vi "Main.vi"(11 "Module Admin":refnum<class "Delacor_lib_QMH_Module Admin.lvclass">) -> ()   [LabVIEW 2020, in "Acquisition.lvlib"]
doc: "This template is based off of the Queued Message Handler design pattern and the Queued Message Handler project template that ships with LabVIEW.\n\nThe main difference is that the queue is private to this module and communication between modules is performed via Broadcast and Request events.\n\nRequest events are wrapped in public API methods and are handled in the Event Handling Loop (EHL) of this VI. Any module can register for Broadcast events sent by this module. The EHL generates messages based on user interface actions.\n\nThe Message Handling Loop (MHL) processes messages generated by the EHL, or by other messages. The messages are string values, so new messages can be added easily to the Message Cases case structure in the MHL. Each message cluster can also provide an optional value for Message Data, which is a variant that can be converted to whatever message-specific data is required.\n_____\nBased on Delacor QMH Project Template 4.0.0.47.\n_____\nBased on DQMH Project Template 6.0.0.91."
uses:
  Acquisition.lvlib
  <vilib>/Delacor/Delacor QMH/Libraries/Module Admin_class/Delacor_lib_QMH_Module Admin.lvclass
  Module Data--cluster.ctl
  CML Shared/Signal Type--enum.ctl
  CML Shared/Calibration Values--cluster.ctl
  Stop Argument--cluster.ctl
  <vilib>/Delacor/Delacor QMH/Libraries/Message Queue_class/Delacor_lib_QMH_Message Queue.lvclass/Delacor_lib_QMH_Message Queue.ctl
  <vilib>/Delacor/Delacor QMH/Libraries/Module Admin_class/Delacor_lib_QMH_Module Admin.lvclass/Delacor_lib_QMH_Module Admin.ctl
  Start Acquiring Argument--cluster.ctl
  Start Acquiring (Reply Payload)--cluster.ctl
  Stop Acquiring Argument--cluster.ctl
  Settings Editor/Update Application Settings (Reply Payload)--cluster.ctl
  Settings Editor/Settings--cluster.ctl
  <vilib>/Utility/miscctls.llb/LVPointTypeDef.ctl
  <vilib>/Delacor/Delacor QMH/Libraries/Message Queue_class/Delacor_lib_QMH_Enqueue Message (Single).vi
  <vilib>/Delacor/Delacor QMH/Libraries/Module Admin_class/Delacor_lib_QMH_Get External Launch.vi
  <vilib>/Utility/error.llb/Error Cluster From Error Code.vi
  <vilib>/ErrorRing/Error Ring.xnode
  <vilib>/Delacor/Delacor QMH/Libraries/Message Queue_class/Delacor_lib_QMH_Message Queue.lvclass
  CML Shared/CML Shared.lvlib
  Settings Editor/Settings Editor.lvlib
  Logger/Logger.lvlib
panel:
  out "Settings":T1
  out "Graph Data":waveform(dbl)[](array[waveform])
  out "error out":errorcluster
  # "This is a headless module. Show its panel to confirm that the Settings are updated correctly and other debugging tasks. Use the Settings Editor to change the settings for this module."
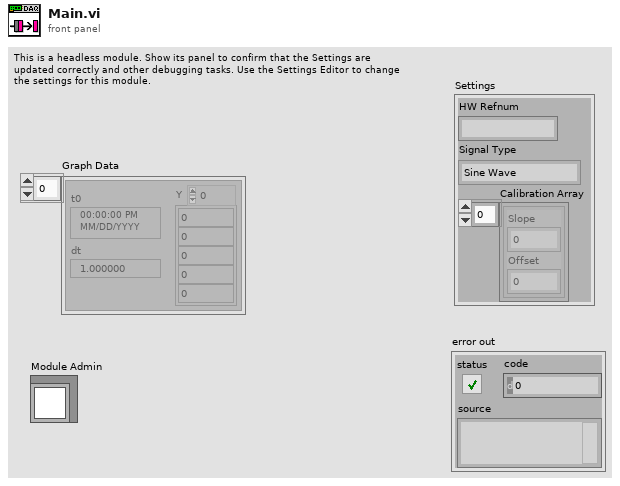
[diagram p1: front panel]
types:
  T1 = typedef "Acquisition.lvlib/Module Data--cluster.ctl" = cluster{"HW Refnum":string, "Signal Type":T2, "Calibration Array":T3[]}
  T2 = typedef "CML Shared.lvlib/Signal Type--enum.ctl" = enum16{"Sine Wave", "Square with Noise"}
  T3 = typedef "CML Shared.lvlib/Calibration Values--cluster.ctl" = cluster{"Slope":dbl, "Offset":dbl}
  T4 = typedef "Settings Editor.lvlib/Broadcast Events--cluster.ctl" = cluster{"Module Did Init":refnum<user-event>, "Status Updated":refnum<user-event>, "Error Reported":refnum<user-event>, "Module Did Stop":refnum<user-event>, "Update Module Execution Status":refnum<user-event>, "Application Settings Updated":refnum<user-event>}
  T5 = typedef "Acquisition.lvlib/Request Events--cluster.ctl" = cluster{"Stop Module":refnum<user-event>, "Show Panel":refnum<user-event>, "Hide Panel":refnum<user-event>, "Get Module Execution Status":refnum<user-event>, "Show Diagram":refnum<user-event>, "Stop Acquiring":refnum<user-event>, "Wakeup Helper Loop":refnum<user-event>, "Change Settings":refnum<user-event>, "Calibrate DAQ":refnum<user-event>, "Start Acquiring":refnum<user-event>}
  T6 = enum32{"invalid lock state", "Not Locked", "Locked (No Password)", "Password-protected"}
  T7 = typedef "Acquisition.lvlib/Stop Argument--cluster.ctl" = cluster{"Origin":string, "Exit via Stop Module Req?":bool, "Wait for Module to stop?":bool}
  T8 = typedef "Acquisition.lvlib/Start Acquiring Argument--cluster.ctl" = cluster{"Wait Notifier":refnum<notifier>, "wait for reply":bool}
  T9 = typedef "Acquisition.lvlib/Stop Acquiring Argument--cluster.ctl" = cluster{"Boolean":bool}
  T10 = typedef "Settings Editor.lvlib/Update Application Settings (Reply Payload)--cluster.ctl" = cluster{"Settings":T11, "Update Settings_error":errorcluster}
  T11 = typedef "Settings Editor.lvlib/Settings--cluster.ctl" = cluster{"Signal Type":T2, "Calibration Array":T3[], "Log File Base Path":path}
  T12 = typedef "LVPointTypeDef.ctl" = cluster{"Horizontal":i16, "Vertical":i16}
  T13 = enum32{"Invalid", "Standard", "Closed", "Hidden", "Minimized", "Maximized"}
  T14 = typedef "Acquisition.lvlib/Start Acquiring (Reply Payload)--cluster.ctl" = cluster{"HW ID":string, "Start Acquiring_error":errorcluster}
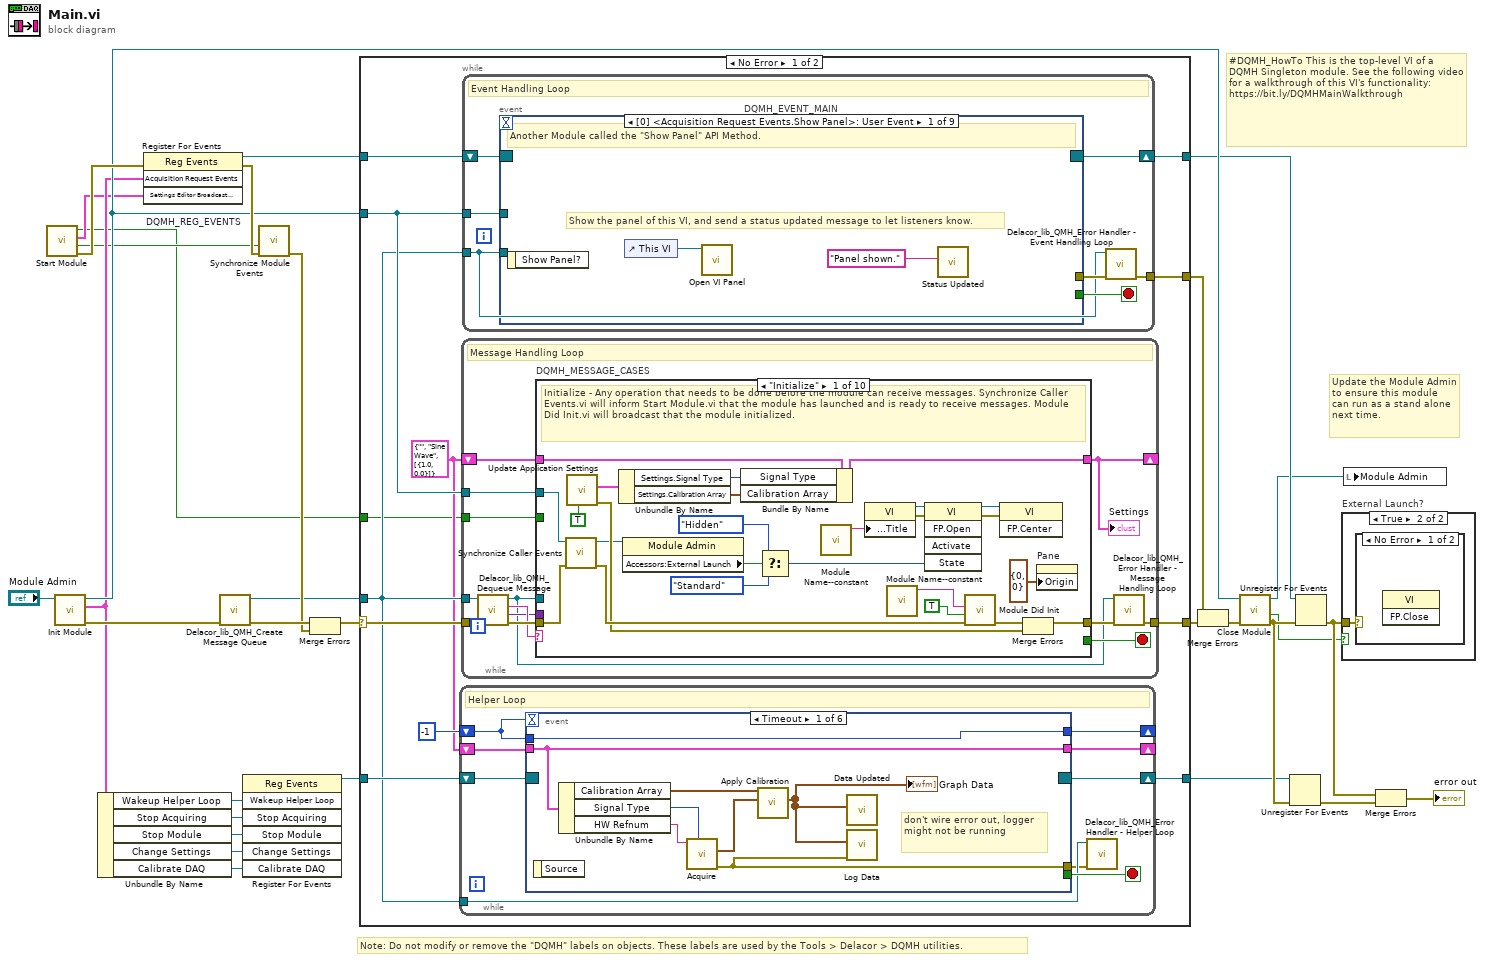
[diagram p0: block diagram]
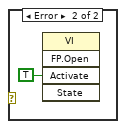
[diagram p3: hidden frame]
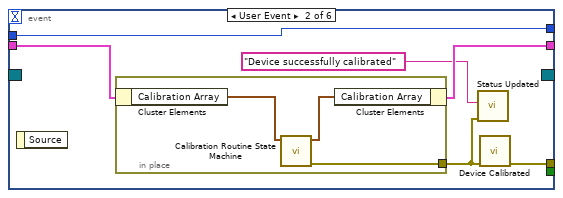
[diagram p4: hidden frame]
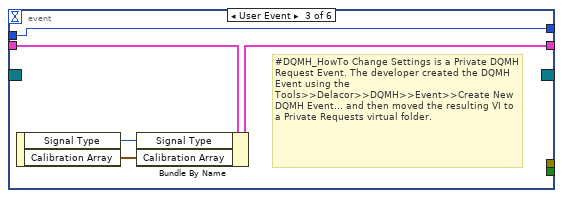
[diagram p5: hidden frame]
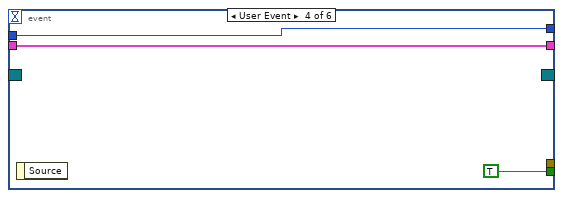
[diagram p6: hidden frame]
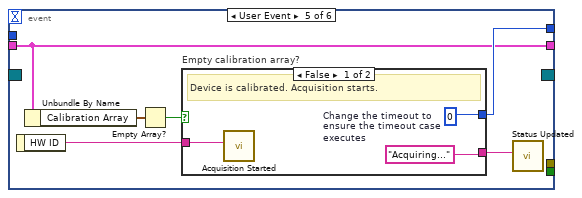
[diagram p7: hidden frame]
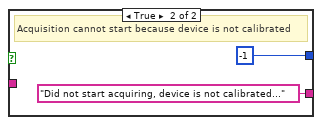
[diagram p8: hidden frame]
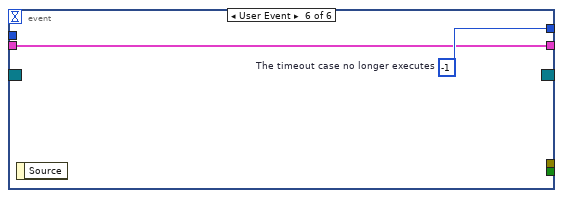
[diagram p9: hidden frame]
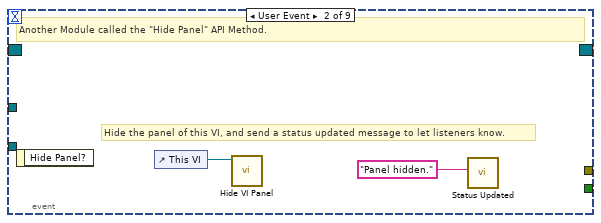
[diagram p10: hidden frame]
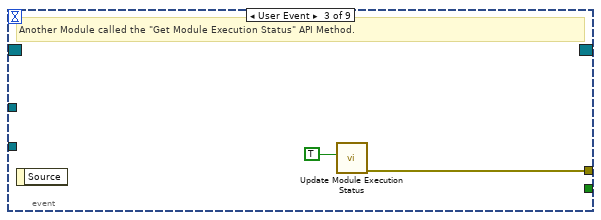
[diagram p11: hidden frame]
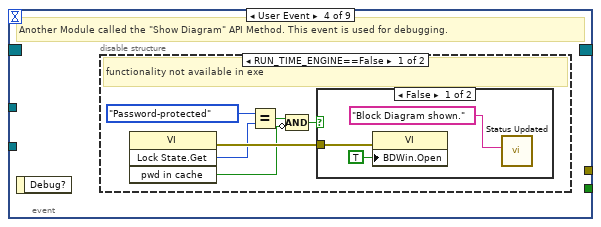
[diagram p12: hidden frame]
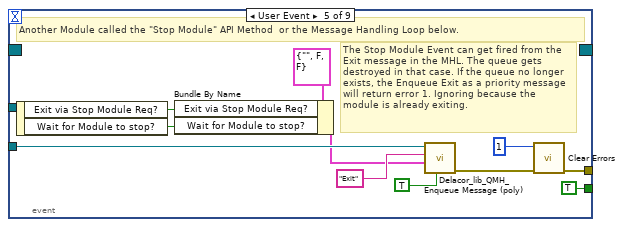
[diagram p15: hidden frame]
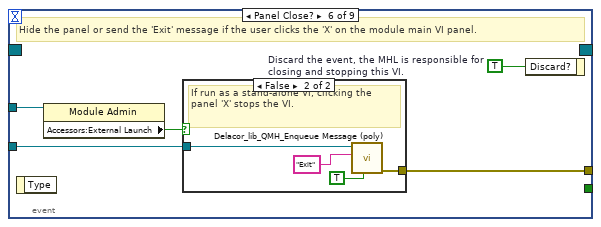
[diagram p16: hidden frame]
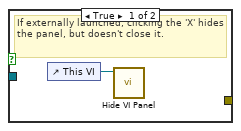
[diagram p17: hidden frame]
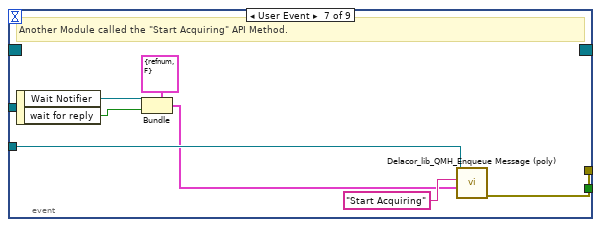
[diagram p18: hidden frame]
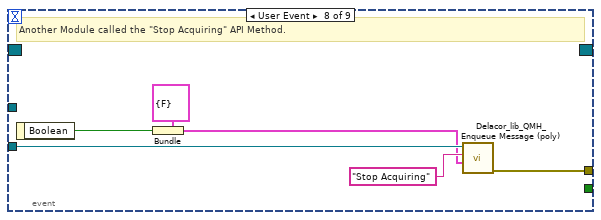
[diagram p19: hidden frame]
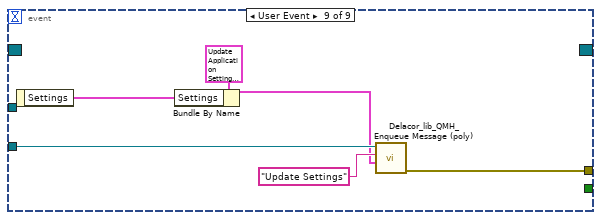
[diagram p20: hidden frame]
diagram:
  # "#DQMH_HowTo This is the top-level VI of a DQMH Singleton module. See the following video for a walkthrough of this VI's functionality: https://bit.ly/DQMHMainWalkthrough"
  # "Note: Do not modify or remove the \"DQMH\" labels on objects. These labels are used by the Tools > Delacor > DQMH utilities."
  # "Update the Module Admin to ensure this module can run as a stand alone next time."
  n1 = call "Start Module.vi"() -> ("error out"=w24:errorcluster, "Wait for Event Sync?"=w5:bool, "Settings Editor Broadcast Events"=w6:T4, "Module Was Already Running?"=w1:bool)  [unwired: 8 in]
  n2 = call "Init Module.vi"("Singleton Module Admin in"="Module Admin") -> ("error out"=w30:errorcluster, "Acquisition Request Events"=w11:T5, "Singleton Module Admin out"=w18:refnum<class "Delacor_lib_QMH_Module Admin.lvclass">)  [unwired: 8 in]
  n3 = Unbundle By Name(w11) -> ("Wakeup Helper Loop"=w7:refnum<user-event>, "Stop Acquiring"=w10:refnum<user-event>, "Stop Module"=w9:refnum<user-event>, "Change Settings"=w4:refnum<user-event>, "Calibrate DAQ"=w3:refnum<user-event>)
  n4 = register-events "DQMH_REG_EVENTS"(error in=w24, w11, w6) -> (reference out=w16:refnum<event-registration>, error out=w23:errorcluster)  [unwired: 1 in]
  n5 = call <vilib>:"Delacor_lib_QMH_Create Message Queue.vi"("error in"=w30) -> ("error out"=w26:errorcluster, "Message Queue"=w15:refnum<class "Delacor_lib_QMH_Message Queue.lvclass">)  [unwired: 9 in]
  n6 = register-events(w7, w10, w9, w4, w3) -> (reference out=w8:refnum<event-registration>)  [unwired: 2 in, 1 out]
  n7 = call "Synchronize Module Events.vi"("error in (no error)"=w23, "Wait for Event Sync?"=w5) -> ("error out"=w22:errorcluster)  [unwired: 9 in]
  n8 = Merge Errors(w26, w22) -> (w25:errorcluster)
  n9 = case shown="No Error" w25 {
    selector: w25 -> [w41 w286]
    tunnel: [w43 w285] -> w31
    tunnel: [w40 w294] -> w17
    tunnel: w16 -> [w39 w294]
    tunnel: w15 -> [w35 w287]
    tunnel: [w42 _] -> w29
    tunnel: w18 -> [w38 w290]
    tunnel: w8 -> [w36 w289]
    tunnel: [w33 w289] -> w2
    tunnel: w1 -> [w32 w288]
    frame No Error {
      w34 = T1 {"HW Refnum"="", "Signal Type"=enum."Sine Wave", "Calibration Array"=[{"Slope"=1.0, "Offset"=0.0}]} ("Data Cluster")
      n10 = while {
        shift-right: [w52] -> _
        shift-left: -1 -> [w51]
        tunnel: w35 -> [w45]
        shift-right: [w48] -> _
        shift-left: w34 -> [w47]
        shift-right: [w46] -> w33
        shift-left: w36 -> [w50]
        stop <- w49 stop-if-true
        # "Helper Loop"
        n11 = event shown="[0] Timeout" {
          selector: w50 -> [_ _ _ _ _ _]
          dyn-events: [_ _ _ _ _ _] -> w46
          timeout: w51 -> [_ _ _ _ _ _]
          tunnel: [w59 w65 w74 w77 w82 w90] -> w52
          tunnel: w51 -> [w59 w65 w74 w77 _ _]
          tunnel: [_ _ _ TRUE _ _] -> w49
          tunnel: [w60 w66 _ _ _ _] -> w44
          tunnel: [w56 w63 w72 w75 w79 w89] -> w48
          tunnel: w47 -> [w56 w64 w73 w75 w79 w89]
          event Timeout {
            # "don't wire error out, logger might not be running"
            n12 = event-data() -> ()  [unwired: 1 in, 1 out]
            n13 = Unbundle By Name(w56) -> ("Calibration Array"=w54:T3[], "Signal Type"=w58:T2, "HW Refnum"=w57:string)
            n14 = call "Acquire.vi"("Signal Type"=w58, "HW ID in"=w57) -> ("error out"=w60:errorcluster, "Graph Data"=w55:waveform(dbl)[])  [unwired: 7 in, 1 out]
            n15 = call "Apply Calibration.vi"("Graph Data"=w55, "Calibration Array"=w54) -> ("Calibrated Data"=w53:waveform(dbl)[])  [unwired: 9 in]
            "Graph Data" <- w53
            n16 = call "Data Updated.vi"("Graph Data"=w53) -> ()  [unwired: 10 in, 1 out]
            n17 = call "Log Data.vi"("error in (no error)"=w60, "Waveforms"=w53) -> ()  [unwired: 9 in, 1 out]
          }
          event User Event {
            n18 = event-data() -> ()  [unwired: 1 in, 1 out]
            n19 = in-place {
              in-place-border: [w69] -> w62
              n20 = in-place-cluster #1(w64) -> ("Calibration Array"=w68:T3[])
              n21 = call "Calibration Routine State Machine.vi"("Calibration Array in"=w68) -> ("error out"=w69:errorcluster, "Calibration Array out"=w67:T3[])  [unwired: 9 in]
              n22 = in-place-cluster #1("Calibration Array"=w67) -> (w63:T1)
            }
            n23 = call "Status Updated.vi"("error in (no error)"=w62, "Status"="Device successfully calibrated") -> ()  [unwired: 9 in, 1 out]
            n24 = call "Device Calibrated.vi"("error in (no error)"=w62) -> ("error out"=w66:errorcluster)  [unwired: 10 in]
          }
          event User Event {
            # "#DQMH_HowTo Change Settings is a Private DQMH Request Event. The developer created the DQMH Event using the Tools>>Delacor>>DQMH>>Event>>Create New DQMH Event... and then moved the resulting VI to a Private Requests virtual folder."
            n25 = event-data() -> ("Signal Type"=w71:T2, "Calibration Array"=w70:T3[])  [unwired: 1 in]
            n26 = Bundle By Name(cluster=w73, "Signal Type"=w71, "Calibration Array"=w70) -> (w72:T1)
          }
          event User Event {
            n27 = event-data() -> ()  [unwired: 1 in, 1 out]
          }
          event User Event {
            n28 = event-data() -> ("HW ID"=w80:string)  [unwired: 1 in]
            n29 = Unbundle By Name(w79) -> ("Calibration Array"=w78:T3[])
            n30 = Empty Array?(array=w78) -> (empty?=w83:bool)
            n31 = case "Empty calibration array?" shown="False" w83 {
              tunnel: ["Acquiring..." ("Status") "Did not start acquiring, device is not calibrated..." ("Status")] -> w81
              tunnel: [w85 -1] -> w82
              tunnel: w80 -> [w86 _]
              frame False {
                w85 = 0  # Change the timeout to ensure the timeout case executes
                # "Device is calibrated. Acquisition starts."
                n32 = call "Acquisition Started.vi"("HW ID"=w86) -> ()  [unwired: 10 in, 1 out]
              }
              frame True {
                # "Acquisition cannot start because device is not calibrated"
              }
            }
            n33 = call "Status Updated.vi"("Status"=w81) -> ()  [unwired: 10 in, 1 out]
          }
          event User Event {
            w90 = -1  # The timeout case no longer executes
            n34 = event-data() -> ()  [unwired: 1 in, 1 out]
          }
        }
        n35 = call-dynamic "Delacor_lib_QMH_Error Handler - Helper Loop.vi"("error in"=w44, "Message Queue in"=w45) -> ()  [unwired: 8 in, 2 out]
      }
      n36 = while {
        tunnel: w35 -> [w156]
        shift-right: [w160] -> _
        shift-left: w34 -> [w161]
        tunnel: w41 -> [w164]
        tunnel: [w162] -> w43
        tunnel: w38 -> [w154]
        tunnel: w32 -> [w153]
        stop <- w159 stop-if-true
        # "Message Handling Loop"
        n37 = call-dynamic "Delacor_lib_QMH_Dequeue Message.vi"("error in"=w164, "Message Queue in"=w156) -> ("error out"=w163:errorcluster, "Message Data"=w157:variant, "Message"=w158:string, "Message Queue out"=w155:refnum<class "Delacor_lib_QMH_Message Queue.lvclass">)  [unwired: 6 in]
        n38 = case "DQMH_MESSAGE_CASES" shown="\"Initialize\"" w158 {
          selector: w158 -> [_ _ _ _ _ _ _ _ _ w272]
          tunnel: w155 -> [_ _ _ _ _ _ _ w237 w261 _]
          tunnel: w163 -> [w188 w192 w205 w219 w229 w232 w234 w244 w268 w275]
          tunnel: [w185 w192 w203 w217 w221 w231 w234 w240 w265 w276] -> w165
          tunnel: w161 -> [w175 w191 w193 w214 w226 w230 w233 w239 w253 w273]
          tunnel: [w170 w191 w201 w214 w226 w230 w233 w239 w253 w273] -> w160
          tunnel: [_ _ _ _ _ _ _ _ w260 _] -> w159
          tunnel: w157 -> [_ _ w200 w216 w227 _ _ w238 w259 _]
          tunnel: w154 -> [w176 _ _ _ _ _ _ w236 w254 _]
          tunnel: w153 -> [_ _ _ _ _ _ _ _ w251 _]
          frame "Initialize" {
            # "Initialize - Any operation that needs to be done before the module can receive messages. Synchronize Caller Events.vi will inform Start Module.vi that the module has launched and is ready to receive messages. Module Did Init.vi will broadcast that the module initialized."
            n39 = call "Synchronize Caller Events.vi"("error in (no error)"=w188, "Singleton Module Admin in"=w176) -> ("error out"=w187:errorcluster, "Singleton Module Admin out"=w172:refnum<class "Delacor_lib_QMH_Module Admin.lvclass">)  [unwired: 8 in]
            n40 = call "Update Application Settings.vi"("wait for reply (T)"=TRUE) -> ("error out"=w184:errorcluster, "Reply Payload"=w169:T10)  [unwired: 8 in, 1 out]
            n41 = Unbundle By Name(w169) -> ("Settings.Signal Type"=w168:T2, "Settings.Calibration Array"=w167:T3[])
            n42 = property class="Module Admin"(reference=w172) -> ("Accessors:External Launch"=w180:bool)  [unwired: 1 in, 2 out]
            n43 = Bundle By Name(cluster=w175, "Signal Type"=w168, "Calibration Array"=w167) -> (w170:T1)
            n44 = Select(t=T13."Hidden" ("State"), s=w180, f=T13."Standard" ("State")) -> (s? t:f=w177:T13)
            n45 = call "Module Name--constant.vi"() -> ("Module Name"=w183:string)  [unwired: 11 in]
            n46 = property class="VI"("Front Panel.Title"=w183) -> (reference out=w182:refnum<vi>, error out=w190:errorcluster)  [unwired: 2 in]
            n47 = call "Module Name--constant.vi"() -> ("Module Name"=w173:string)  [unwired: 11 in]
            n48 = invoke class="VI" method="FP.Open"(reference=w182, error in=w190, "State"=w177) -> (reference out=w181:refnum<vi>, error out=w189:errorcluster)  [unwired: 2 in, 3 out]
            n49 = call "Module Did Init.vi"("error in (no error)"=w187, "Initialized?"=TRUE, "Origin"=w173) -> ("error out"=w186:errorcluster)  [unwired: 8 in]
            n50 = invoke class="VI" method="FP.Center"(reference=w181, error in=w189) -> ()  [unwired: 1 in, 3 out]
            n51 = Merge Errors(w186, w184) -> (w185:errorcluster)
            n52 = property on="Pane" class="Pane"("Origin"=T12 {"Horizontal"=0, "Vertical"=0}) -> ()  [unwired: 2 in, 2 out]
          }
          frame "---Module Specific---" {
            # "Separator -- The following cases handle messages specific to this Module."
          }
          frame "Start Acquiring" {
            # "Requests Acquisition Module to start acquiring."
            n53 = Variant To Data(error in=w205, type=T8 {"Wait Notifier"=refnum, "wait for reply"=FALSE} ("Start Acquisition Argument"), Variant=w200) -> (data=w198:T8, error out=w202:errorcluster)
            n54 = in-place {
              in-place-border: [w211] -> w204
              in-place-border: w202 -> [w210]
              in-place-border: [w206] -> w194
              n55 = in-place-cluster #2(w193) -> ("HW Refnum"=w207:string)
              n56 = call "Initialize Hardware References.vi"("error in (no error)"=w210, "HW Refnum in"=w207) -> ("error out"=w209:errorcluster, "HW Refnum out"=w208:string)  [unwired: 8 in]
              n57 = call "Configure Hardware.vi"("error in (no error)"=w209, "HW Refnum in"=w208) -> ("error out"=w211:errorcluster, "HW Refnum out"=w206:string)  [unwired: 8 in]
              n58 = in-place-cluster #2("HW Refnum"=w206) -> (w201:T1)
            }
            n59 = Bundle By Name(cluster=T14 {"HW ID"="", "Start Acquiring_error"={"status"=FALSE, "code"=0, "source"=""}} ("Start Acquisition (Reply Payload)"), "HW ID"=w194, "Start Acquiring_error"=w204) -> (w196:T14)
            n60 = Unbundle By Name(w198) -> ("Wait Notifier"=w197:refnum<notifier>)
            n61 = call "Wakeup Helper Loop.vi"("error in (no error)"=w204, "HW ID"=w194) -> ("error out"=w203:errorcluster)  [unwired: 9 in]
            n62 = Send Notification(notification=w196, notifier=w197) -> ()  [unwired: 1 in, 2 out]
          }
          frame "Stop Acquiring" {
            # "Requests the Acquisition Module to stop acquiring"
            n63 = Variant To Data(error in=w219, type=T9 {"Boolean"=FALSE} ("Stop Acquiring Argument"), Variant=w216) -> (error out=w218:errorcluster)  [unwired: 1 out]
            n64 = Unbundle By Name(w214) -> ("HW Refnum"=w213:string)
            n65 = call "Stop Acquisition.vi"("error in (no error)"=w218, "HW Refnum"=w213) -> ("error out"=w217:errorcluster)  [unwired: 9 in]
            n66 = call "Acquisition Stopped.vi"("error in (no error)"=w217) -> ()  [unwired: 10 in, 1 out]
            n67 = call "Status Updated.vi"("error in (no error)"=w217, "Status"="Acquisition Stopped") -> ()  [unwired: 9 in, 1 out]
          }
          frame "Update Settings" {
            # "Send the Change Settings event to the helper loop."
            # "The Settings Editor broadcasted that the settings have changed."
            n68 = Variant To Data(error in=w229, type=T10 {"Settings"={"Signal Type"=enum."Sine Wave", "Calibration Array"=[], "Log File Base Path"=path ""}, "Update Settings_error"={"status"=FALSE, "code"=0, "source"=""}} ("Settings Updated Argument"), Variant=w227) -> (data=w224:T10, error out=w228:errorcluster)
            n69 = Unbundle By Name(w224) -> ("Settings.Signal Type"=w223:T2, "Settings.Calibration Array"=w222:T3[])
            n70 = call "Change Settings.vi"("error in (no error)"=w228, "Calibration Array"=w222, "Signal Type"=w223) -> ("error out"=w221:errorcluster)  [unwired: 8 in]
            n71 = call "Status Updated.vi"("error in (no error)"=w221, "Status"="Settings Updated") -> ()  [unwired: 9 in, 1 out]
          }
          frame "---Copy This Frame---" {
            # "Duplicate this frame when creating new messages.  Change this comment in the duplicated frame to describe this message."
            n72 = Merge Errors(w232) -> (w231:errorcluster)
          }
          frame "---Exit and Error Handling---" {
            # "Separator - The following cases handle errors and exit messages."
          }
          frame "Error" {
            # "Error - Check the error message data and respond accordingly. This message is sent by the \"Error Handler\" VIs at the end of each loop in this application."
            n73 = property class="Module Admin"(reference=w236) -> ("Accessors:External Launch"=w235:bool)  [unwired: 1 in, 2 out]
            n74 = Variant To Data(error in=w244, type=errorcluster {"status"=FALSE, "code"=0, "source"=""} ("error constant"), Variant=w238) -> (data=w245:errorcluster, error out=w242:errorcluster)
            n75 = call "Error Reported.vi"("Error"=w245) -> ()  [unwired: 10 in, 1 out]
            n76 = case shown="False" w235 {
              tunnel: [w250 _] -> w241
              tunnel: w237 -> [w248 _]
              tunnel: w245 -> [w249 _]
              frame False {
                # "If the module is running standalone, then pop up an error dialog and call the \"Exit\" message."
                n77 = call <vilib>:"Simple Error Handler.vi"("error in (no error)"=w249) -> ()  [unwired: 4 in, 5 out]
                n78 = call-poly <vilib>:"Delacor_lib_QMH_Enqueue Message (poly).vi"("Priority Message? (F)"=TRUE, "Message"="Exit", "Message Queue in"=w248) -> ("error out"=w250:errorcluster)  [unwired: 7 in, 1 out]
              }
              frame True {
                # "If the module was launched externally, calling the Error Reported broadcast VI is the only action performed by the \"Error\" message. The module's caller can then process the error appropriately."
              }
            }
            n79 = Merge Errors(w242, w241) -> (w240:errorcluster)
            n80 = local write "error out"(w240) -> ()
          }
          frame "Exit" {
            w258 = 91  # 91: not all Exit messages will have an argument
            w260 = TRUE  # Stop the VI
            # "Release the message queue reference"
            # "Exit - Exit the application."
            n81 = Variant To Data(error in=w268, type=T7 {"Origin"="", "Exit via Stop Module Req?"=FALSE, "Wait for Module to stop?"=FALSE} ("Stop Argument"), Variant=w259) -> (data=w256:T7, error out=w264:errorcluster)
            n82 = call <vilib>:"Clear Errors.vi"("error in (no error)"=w264, "specific error code to clear (0: all)"=w258) -> ("error out"=w267:errorcluster)  [unwired: 4 in, 1 out]
            n83 = Unbundle By Name(w253) -> ("HW Refnum"=w252:string)
            n84 = control-ref of="This VI"() -> (w255:refnum<vi>)
            n85 = call "Handle Exit.vi"("Stop Argument"=w256, "Admin in"=w254, "VI reference"=w255) -> ("error out"=w263:errorcluster)  [unwired: 7 in, 1 out]
            n86 = call "Close Hardware References.vi"("HW Refnum in"=w252) -> ("error out"=w262:errorcluster)  [unwired: 9 in, 1 out]
            n87 = call-dynamic "Delacor_lib_QMH_Release Message Queue.vi"("error in"=w267, "Message Queue"=w261) -> ("error out"=w266:errorcluster)  [unwired: 9 in]
            n88 = case "Settings Editor was\nalready running?" shown="False" w251 {
              frame False {
                n89 = call "Module Name--constant.vi"() -> ("Module Name"=w270:string)  [unwired: 11 in]
                n90 = call "Stop Module.vi"("Wait for Module to Stop? (F)"=TRUE, "Origin"=w270) -> ()  [unwired: 9 in, 1 out]
              }
              frame True {
                # "Another Module is\nin charge of stopping Settings Editor"
              }
            }
            n91 = Merge Errors(w266, w263, w262) -> (w265:errorcluster)
          }
          frame Default {
            # "'Default' case only runs if there is a message that isn't defined in any of the other cases.  Output a programming error."
            n92 = call "Module Name--constant.vi"() -> ("Module Name"=w271:string)  [unwired: 11 in]
            n93 = xnode "Error Ring"("parameter 0"=w272, "parameter 1"=w271) -> ("error out"=w274:errorcluster)
            n94 = Merge Errors(w275, w274) -> (w276:errorcluster)
          }
        }
        "Settings" <- w160
        n95 = call-dynamic "Delacor_lib_QMH_Error Handler - Message Handling Loop.vi"("error in"=w165, "Message Queue in"=w155) -> ("dup error in"=w162:errorcluster)  [unwired: 8 in, 1 out]
      }
      n96 = while {
        tunnel: w35 -> [w91]
        shift-right: [w94] -> w40
        shift-left: w39 -> [w95]
        tunnel: [w96] -> w42
        tunnel: w38 -> [w92]
        stop <- w93 stop-if-true
        # "Event Handling Loop"
        n97 = event "DQMH_EVENT_MAIN" shown="[0] <Acquisition Request Events.Show Panel>: User Event" {
          selector: w95 -> [_ _ _ _ _ _ _ _ _]
          dyn-events: [_ _ _ _ _ _ _ _ _] -> w94
          timeout: _ -> [_ _ _ _ _ _ _ _ _]
          tunnel: [_ _ _ _ TRUE ("Discard?") _ _ _ _] -> w93
          tunnel: w91 -> [_ _ _ _ w119 w126 w140 w145 w150]
          tunnel: [_ _ w103 _ w122 w128 w136 w146 w152] -> w97
          tunnel: w92 -> [_ _ _ _ _ w125 _ _ _]
          event User Event {
            # "Show the panel of this VI, and send a status updated message to let listeners know."
            # "Another Module called the \"Show Panel\" API Method."
            n98 = event-data() -> ()  [unwired: 1 in, 1 out]
            n99 = control-ref of="This VI"() -> (w99:refnum<vi>)
            n100 = call "Open VI Panel.vi"("VI"=w99) -> ()  [unwired: 10 in, 1 out]
            n101 = call "Status Updated.vi"("Status"="Panel shown." ("format string")) -> ()  [unwired: 10 in, 1 out]
          }
          event User Event {
            # "Hide the panel of this VI, and send a status updated message to let listeners know."
            # "Another Module called the \"Hide Panel\" API Method."
            n102 = event-data() -> ()  [unwired: 1 in, 1 out]
            n103 = control-ref of="This VI"() -> (w101:refnum<vi>)
            n104 = call "Hide VI Panel.vi"("VI"=w101) -> ()  [unwired: 10 in, 1 out]
            n105 = call "Status Updated.vi"("Status"="Panel hidden." ("format string")) -> ()  [unwired: 10 in, 1 out]
          }
          event User Event {
            # "Another Module called the \"Get Module Execution Status\" API Method."
            n106 = event-data() -> ()  [unwired: 1 in, 1 out]
            n107 = call "Update Module Execution Status.vi"("Running?"=TRUE) -> ("error out"=w103:errorcluster)  [unwired: 10 in]
          }
          event User Event {
            # "Another Module called the \"Show Diagram\" API Method. This event is used for debugging."
            n108 = event-data() -> ()  [unwired: 1 in, 1 out]
            n109 = disable-structure shown="RUN_TIME_ENGINE==False" {
              frame condition #0 (active) {
                # "functionality not available in exe"
                n110 = invoke class="VI" method="Lock State.Get"() -> (error out=w109:errorcluster, "Get Lock State"=w108:T6, "pwd in cache"=w105:bool)  [unwired: 4 in, 1 out]
                n111 = Equal?(x=T6."Password-protected", y=w108) -> (x = y?=w106:bool)
                n112 = Compound Arithmetic op=AND(w106, invert w105) -> (w104:bool)
                n113 = case shown="False" w104 {
                  tunnel: w109 -> [w112 _]
                  frame False {
                    n114 = property class="VI"(error in=w112, "BDWin.Open"=TRUE ("Block Diagram Window:Open")) -> ()  [unwired: 1 in, 2 out]
                    n115 = call "Status Updated.vi"("Status"="Block Diagram shown." ("format string")) -> ()  [unwired: 10 in, 1 out]
                  }
                  frame True {
                    # "Password-protected VI, and the password is not in the cache. Do not show the diagram."
                  }
                }
              }
              frame condition #1 {
              }
            }
          }
          event User Event {
            # "The Stop Module Event can get fired from the Exit message in the MHL. The queue gets destroyed in that case. If the queue no longer exists, the Enqueue Exit as a priority message will return error 1. Ignoring because the module is already exiting."
            # "Another Module called the \"Stop Module\" API Method  or the Message Handling Loop below."
            n116 = event-data() -> ("Exit via Stop Module Req?"=w115:bool, "Wait for Module to stop?"=w114:bool)  [unwired: 1 in]
            n117 = Bundle By Name(cluster=T7 {"Origin"="", "Exit via Stop Module Req?"=FALSE, "Wait for Module to stop?"=FALSE} ("Stop Argument"), "Exit via Stop Module Req?"=w115, "Wait for Module to stop?"=w114) -> (w113:T7)
            n118 = call-poly <vilib>:"Delacor_lib_QMH_Enqueue Message (poly).vi"("Priority Message? (F)"=TRUE, "Message Data"=w113, "Message"="Exit", "Message Queue in"=w119) -> ("error out"=w123:errorcluster)  [unwired: 6 in, 1 out]
            n119 = call <vilib>:"Clear Errors.vi"("error in (no error)"=w123, "specific error code to clear (0: all)"=1) -> ("error out"=w122:errorcluster)  [unwired: 4 in, 1 out]
          }
          event Panel Close? {
            w127 = TRUE  # Discard the event, the MHL is responsible for closing and stopping this VI.
            # "Hide the panel or send the 'Exit' message if the user clicks the 'X' on the module main VI panel."
            n120 = event-data() -> ()  [unwired: 1 in, 1 out]
            n121 = property class="Module Admin"(reference=w125) -> ("Accessors:External Launch"=w124:bool)  [unwired: 1 in, 2 out]
            n122 = case shown="False" w124 {
              tunnel: w126 -> [_ w132]
              tunnel: [_ w133] -> w128
              frame True {
                # "If externally launched, clicking the 'X' hides the panel, but doesn't close it."
                n123 = control-ref of="This VI"() -> (w129:refnum<vi>)
                n124 = call "Hide VI Panel.vi"("VI"=w129) -> ()  [unwired: 10 in, 1 out]
              }
              frame False {
                # "If run as a stand-alone VI, clicking the panel 'X' stops the VI."
                n125 = call-poly <vilib>:"Delacor_lib_QMH_Enqueue Message (poly).vi"("Priority Message? (F)"=TRUE, "Message"="Exit", "Message Queue in"=w132) -> ("error out"=w133:errorcluster)  [unwired: 7 in, 1 out]
              }
            }
            n126 = event-data("Discard?"=w127) -> ()  [unwired: 1 in, 1 out]
          }
          event User Event {
            # "Another Module called the \"Start Acquiring\" API Method."
            n127 = event-data() -> ("Wait Notifier"=w135:refnum<notifier>, "wait for reply"=w134:bool)  [unwired: 1 in]
            n128 = Bundle(cluster=T8 {"Wait Notifier"=refnum, "wait for reply"=FALSE} ("Start Acquisition Argument"), "Wait Notifier"=w135, "wait for reply"=w134) -> (w137:T8)
            n129 = call-poly <vilib>:"Delacor_lib_QMH_Enqueue Message (poly).vi"("Message Data"=w137, "Message"="Start Acquiring", "Message Queue in"=w140) -> ("error out"=w136:errorcluster)  [unwired: 7 in, 1 out]
          }
          event User Event {
            # "Another Module called the \"Stop Acquiring\" API Method."
            n130 = event-data() -> ("Boolean"=w141:bool)  [unwired: 1 in]
            n131 = Bundle(cluster=T9 {"Boolean"=FALSE} ("Stop Acquiring Argument"), "Boolean"=w141) -> (w142:T9)
            n132 = call-poly <vilib>:"Delacor_lib_QMH_Enqueue Message (poly).vi"("Message Data"=w142, "Message"="Stop Acquiring", "Message Queue in"=w145) -> ("error out"=w146:errorcluster)  [unwired: 7 in, 1 out]
          }
          event User Event {
            n133 = event-data() -> ("Settings"=w147:T11)  [unwired: 1 in]
            n134 = Bundle By Name(cluster=T10 {"Settings"={"Signal Type"=enum."Sine Wave", "Calibration Array"=[], "Log File Base Path"=path ""}, "Update Settings_error"={"status"=FALSE, "code"=0, "source"=""}} ("Settings Updated Argument"), "Settings"=w147) -> (w149:T10)
            n135 = call-poly <vilib>:"Delacor_lib_QMH_Enqueue Message (poly).vi"("Message Data"=w149, "Message"="Update Settings", "Message Queue in"=w150) -> ("error out"=w152:errorcluster)  [unwired: 7 in, 1 out]
          }
        }
        n136 = call-dynamic "Delacor_lib_QMH_Error Handler - Event Handling Loop.vi"("error in"=w97, "Message Queue in"=w91) -> ("dup error in"=w96:errorcluster)  [unwired: 8 in, 1 out]
      }
    }
    frame Error {
      # "Synchronize Caller Events.vi will inform Start Module.vi that the module has launched and will let the code calling Start Module.vi register for broadcasts and would permit the caller receive the broadcast that an error occurred at launch time."
      n137 = call "Synchronize Caller Events.vi"("Singleton Module Admin in"=w290) -> ("error out"=w295:errorcluster)  [unwired: 9 in, 1 out]
      n138 = call-dynamic "Delacor_lib_QMH_Release Message Queue.vi"("error in"=w286, "Message Queue"=w287) -> ("error out"=w285:errorcluster)  [unwired: 9 in]
      n139 = call "Module Name--constant.vi"() -> ("Module Name"=w293:string)  [unwired: 11 in]
      n140 = case "Settings Editor was\nalready running?" shown="False" w288 {
        frame False {
          n141 = call "Module Name--constant.vi"() -> ("Module Name"=w298:string)  [unwired: 11 in]
          n142 = call "Stop Module.vi"("Wait for Module to Stop? (F)"=TRUE, "Origin"=w298) -> ()  [unwired: 9 in, 1 out]
        }
        frame True {
          # "Another Module is\nin charge of stopping Settings Editor"
        }
      }
      n143 = Format Into String(format string="An error occurred during initialization. %s is no longer running.", w293) -> (resulting string=w291:string)  [unwired: 2 in, 1 out]
      n144 = Merge Errors(w285, w295) -> (w296:errorcluster)
      n145 = call "Error Reported.vi"("Additional Information"=w291, "Error"=w296) -> ()  [unwired: 9 in, 1 out]
    }
  }
  n146 = Merge Errors(w29, w31) -> (w28:errorcluster)
  n147 = call "Close Module.vi"("error in (no error)"=w28, "Module Admin in"=w18) -> ("error out"=w21:errorcluster, "External Launch"=w12:bool, "Module Admin out"=w13:refnum<class "Delacor_lib_QMH_Module Admin.lvclass">)  [unwired: 7 in]
  n148 = Unregister For Events(event registration refnum=w2, error in=w21) -> (error out=w19:errorcluster)
  n149 = Unregister For Events(event registration refnum=w17, error in=w21) -> (error out=w27:errorcluster)
  n150 = case "External Launch?" shown="True" w12 {
    tunnel: w27 -> [_ w299]
    frame False {
    }
    frame True {
      n151 = case shown="No Error" w299 {
        frame No Error {
          n152 = invoke class="VI" method="FP.Close"() -> ()  [unwired: 3 in, 3 out]
        }
        frame Error {
          n153 = invoke class="VI" method="FP.Open"("Activate"=TRUE ("Activate?")) -> ()  [unwired: 4 in, 5 out]
        }
      }
    }
  }
  n154 = local write "Module Admin"(w13) -> ()
  n155 = Merge Errors(w27, w19) -> (→"error out":errorcluster)
